vi "automatic_steps_write.vi"(7 "references":T1, 8 "error in (no error)":errorcluster, 11 "automatic_steps":variant) -> (0 "error out":errorcluster, 3 "automatic_steps_replaced":bool)   [LabVIEW 2015, in "lv-recipe-machine.lvlib"]
uses:
  lv-recipe-machine.lvlib
  _controls/references.ctl
  _controls/input.ctl
  _controls/input_command.ctl
  _controls/output.ctl
  _controls/data.ctl
  _controls/configuration.ctl
  _controls/recipe_data.ctl
  _controls/mode.ctl
  _controls/manual_state.ctl
  _controls/automatic_state.ctl
  _controls/recipe_step.ctl
  <userlib>/antonio-alexander/lv-waitgroup/public/_controls/api_waitgroup.ctl
  _controls/change.ctl
  _controls/status.ctl
  <userlib>/antonio-alexander/lv-waitgroup/lv-waitgroup.lvlib
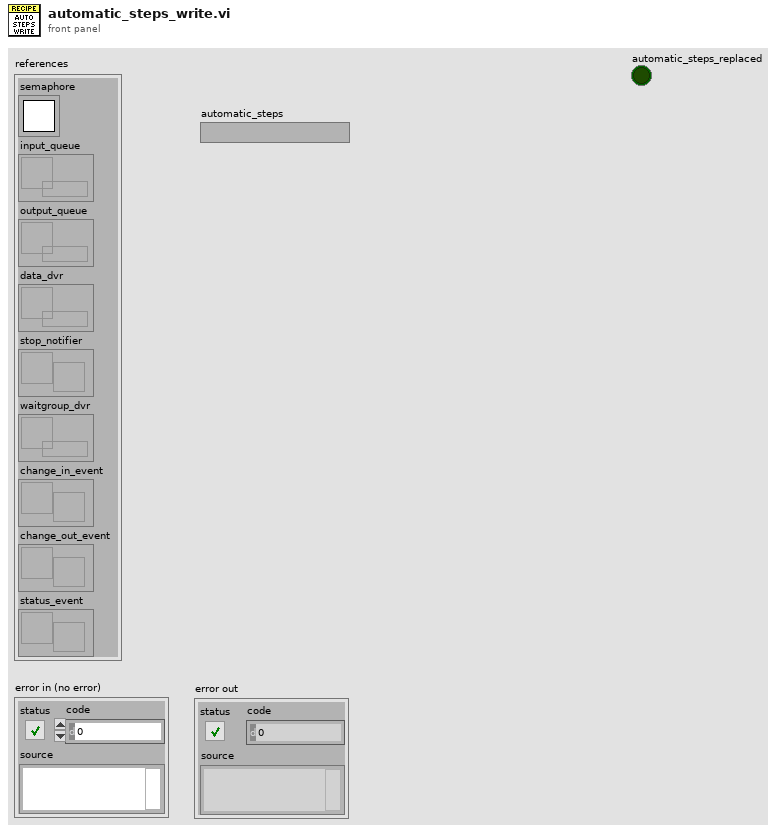
[diagram p1: front panel]
types:
  T1 = typedef "lv-recipe-machine.lvlib/references.ctl" = cluster{"semaphore":T2, "input_queue":refnum<queue>, "output_queue":refnum<queue>, "data_dvr":refnum<data-value>, "stop_notifier":refnum<notifier>, "waitgroup_dvr":refnum<data-value>, "change_in_event":refnum<user-event>, "change_out_event":refnum<user-event>, "status_event":refnum<user-event>}
  T2 = typedef "Semaphore RefNum" = refnum<k1>
  T3 = typedef "lv-recipe-machine.lvlib/data.ctl" = cluster{"configuration":T4, "working":cluster{"recipe_data":T5, "api_waitgroup":T10}}
  T4 = typedef "lv-recipe-machine.lvlib/configuration.ctl" = cluster{dbl}
  T5 = typedef "lv-recipe-machine.lvlib/recipe_data.ctl" = cluster{"mode":T6, "manual_state":T7, "automatic_state":T8, "manual":cluster{"step_action":string, "data":variant, "actions":variant}, "automatic":cluster{"data":variant, "steps":variant, "criteria":variant, "index":i32, "recipe []":T9[]}}
  T6 = typedef "lv-recipe-machine.lvlib/mode.ctl" = enum16{"<mode>", "manual", "automatic", "<null>"}
  T7 = typedef "lv-recipe-machine.lvlib/manual_state.ctl" = enum16{"<manual_state>", "failed", "action", "running", "idle", "<null>"}
  T8 = typedef "lv-recipe-machine.lvlib/automatic_state.ctl" = enum16{"<automatic_state>", "failed", "idle", "running", "paused", "transition", "stopped", "<null>"}
  T9 = typedef "lv-recipe-machine.lvlib/recipe_step.ctl" = cluster{"step":string, "data":variant}
  T10 = typedef "lv-waitgroup.lvlib/api_waitgroup.ctl" = cluster{"waitgroups":refnum<data-value>, "waitgroup":string}
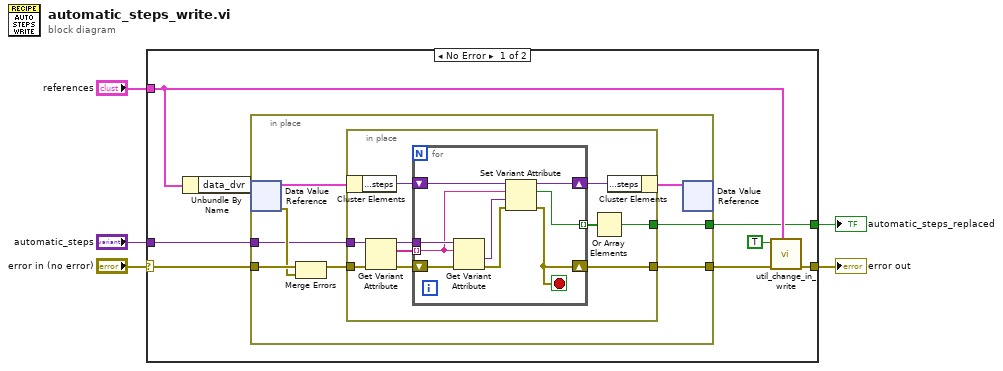
[diagram p0: block diagram]
diagram:
  n1 = case shown="No Error" "error in (no error)" {
    selector: "error in (no error)" -> [w12 w41]
    tunnel: [w10 w41] -> w2
    tunnel: "references" -> [w11 _]
    tunnel: "automatic_steps" -> [w9 _]
    tunnel: [w6 _] -> w1
    frame No Error {
      n2 = Unbundle By Name(w11) -> ("data_dvr"=w13:refnum<data-value>)
      n3 = in-place {
        in-place-border: [w15] -> w8
        in-place-border: w12 -> [w21]
        in-place-border: w9 -> [w17]
        in-place-border: [w14] -> w6
        n4 = in-place-dvr #1(w13) -> (w19:T3, w20:errorcluster)
        n5 = Merge Errors(w21, w20) -> (w16:errorcluster)
        n6 = in-place {
          in-place-border: w17 -> [w29]
          in-place-border: w16 -> [w28]
          in-place-border: [w24] -> w15
          in-place-border: [w22] -> w14
          n7 = in-place-cluster #2(w19) -> ("working.recipe_data.automatic.steps"=w31:variant)
          n8 = Get Variant Attribute(Variant=w29, error in=w28) -> (duplicate Variant=w27:variant, names=w26:string[], error out=w25:errorcluster)  [unwired: 2 in, 1 out]
          n9 = for {
            shift-right: [w39] -> w30
            shift-left: w31 -> [w40]
            tunnel: [w38] -> w23 mode=indexing
            tunnel: w27 -> [w36]
            tunnel: w26 -> [w32] mode=indexing
            shift-right: [w37] -> w24
            shift-left: w25 -> [w35]
            stop <- w37 stop-if-true
            n10 = Get Variant Attribute(Variant=w36, name=w32, error in=w35) -> (value=w33:variant, error out=w34:errorcluster)  [unwired: 1 in, 2 out]
            n11 = Set Variant Attribute(Variant=w40, name=w32, value=w33, error in=w34) -> (Variant out=w39:variant, replaced=w38:bool, error out=w37:errorcluster)
          }
          n12 = Or Array Elements(Boolean array=w23) -> (logical OR=w22:bool)
          n13 = in-place-cluster #2("working.recipe_data.automatic.steps"=w30) -> (w18:T3)
        }
        n14 = in-place-dvr #1(w18) -> ()  [unwired: 2 out]
      }
      n15 = call "util_change_in_write.vi"("references"=w11, "error in (no error)"=w8, "data"=TRUE ("change")) -> ("error out"=w10:errorcluster)  [unwired: 8 in]
    }
    frame Error {
    }
  }
  "error out" <- w2
  "automatic_steps_replaced" <- w1
